vi "PV HLT5xx Control mode.vi"(7 "Adress of unit":u16=1 min=1 max=999 step=1, 8 "error in (no error)":errorcluster, 9 "set control mode":u16(ring)=4 items=["Local", "RS232 / RS485", "SPS", "Local, RS232 / RS485", "All (default)"], 10 "Parameter\nread only<->describe":bool, 11 "VISA session":refnum<visa-resource-name>) -> (0 "error out":errorcluster, 1 "control mode out":u16(ring)=4 items=["Local", "RS232 / RS485", "SPS", "Local, RS232 / RS485", "All (default)"], 2 "response (data)":string, 3 "dup VISA session":refnum<visa-resource-name>)   [LabVIEW 2021, in "Pfeiffer Vacuum.lvlib"]
doc: "This VI allows you to set or check the \"Control Mode (Para 604)\" on the SmartTest (HLT5xx)."
uses:
  <instrlib>/Pfeiffer Vacuum/Pfeiffer Vacuum.lvlib
panel:
  # "Control mode"
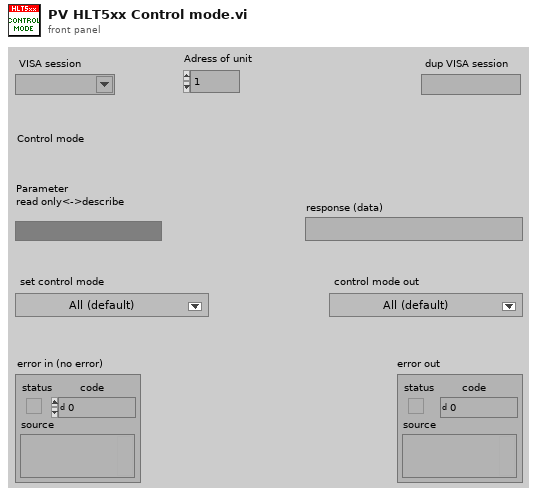
[diagram p1: front panel]
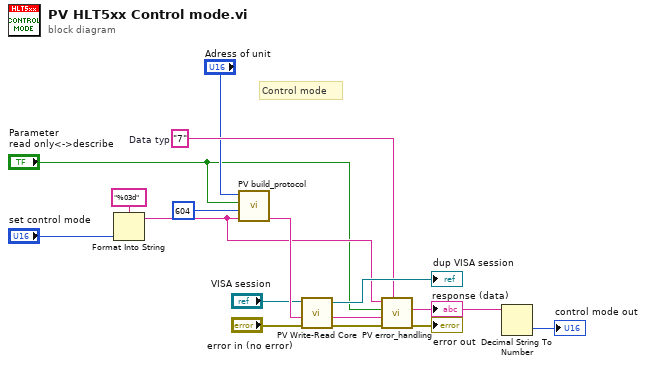
[diagram p0: block diagram]
diagram:
  w10 = "7"  # Data typ
  # "Control mode"
  n1 = Format Into String(format string="%03d" ("Format-String"), "set control mode") -> (resulting string=w11:string)  [unwired: 2 in, 1 out]
  n2 = call <instrlib>:"PV build_protocol.vi"("Data"=w11, "Parameter-number"=u16 604, "parameter\nread<->describe"="Parameter\nread only<->describe", "Adress"="Adress of unit") -> ("output"=w15:string)  [unwired: 3 in]
  n3 = call <instrlib>:"PV Write-Read Core.vi"("error in"="error in (no error)", "Write data in"=w15, "VISA session"="VISA session") -> ("error out"=w13:errorcluster, "response (data) out"=w14:string, "dup VISA session"=→"dup VISA session":refnum<visa-resource-name>)  [unwired: 2 in]
  n4 = call <instrlib>:"PV error_handling.vi"("Data Typ in"=w10, "error in"=w13, "response (data) in"=w14, "Parameter\nread only<->describe"="Parameter\nread only<->describe", "data in"=w11) -> ("error out"=→"error out":errorcluster, "Data out"=w8:string)  [unwired: 4 in, 1 out]
  "response (data)" <- w8
  n5 = Decimal String To Number(string=w8) -> (number=→"control mode out":i32)  [unwired: 2 in, 1 out]
